vi "CHS_Teleop_System_CalcDriveMode.vi"(4 "Abs Traj 2":bool, 6 "Abs Traj 1":bool, 8 "Traj Rev Follow Orient":bool, 9 "Traj Rev Same Orient":bool, 10 "Traj Fwd Follow Orient":bool, 11 "Traj Fwd Same Orient":bool) -> (2 "Dirve Mode Changed":bool, 3 "Drive Mode":i32)   [LabVIEW 2019]
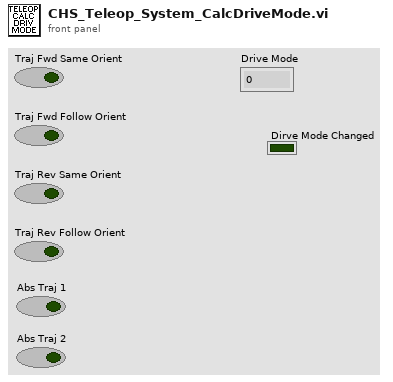
[diagram p1: front panel]
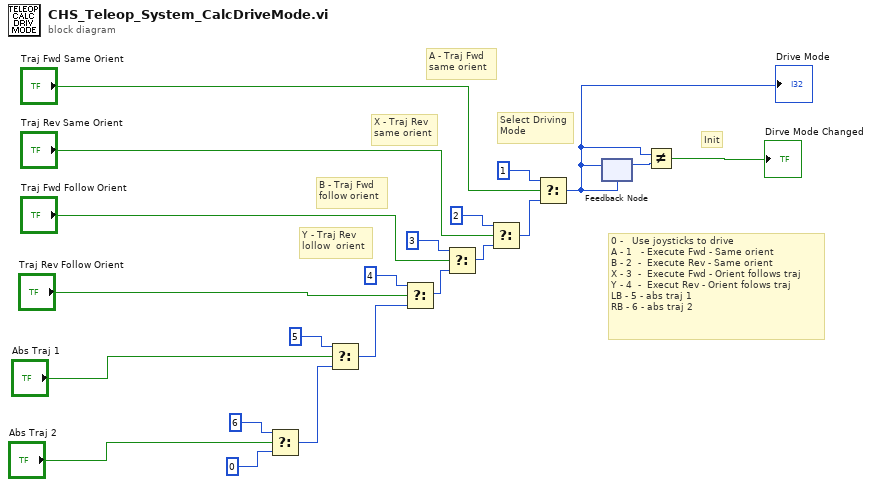
[diagram p0: block diagram]
diagram:
  # "0 -   Use joysticks to drive\nA - 1   - Execute Fwd - Same orient\nB - 2  -  Execute Rev - Same orient\nX - 3  -  Execute Fwd - Orient follows traj\nY - 4  -  Execut Rev - Orient folows traj\nLB - 5 - abs traj 1\nRB - 6 - abs traj 2"
  # "Init"
  # "Y - Traj Rev \nlollow  orient"
  # "B - Traj Fwd \nfollow orient"
  # "X - Traj Rev\nsame orient"
  # "A - Traj Fwd \nsame orient"
  # "Select Driving\nMode"
  n1 = Select(t=6, s="Abs Traj 2", f=0) -> (s? t:f=w3:i32)
  n2 = Select(t=5, s="Abs Traj 1", f=w3) -> (s? t:f=w4:i32)
  n3 = Select(t=4, s="Traj Rev Follow Orient", f=w4) -> (s? t:f=w18:i32)
  n4 = Select(t=3, s="Traj Fwd Follow Orient", f=w18) -> (s? t:f=w17:i32)
  n5 = Select(t=2, s="Traj Rev Same Orient", f=w17) -> (s? t:f=w14:i32)
  n6 = Select(t=1, s="Traj Fwd Same Orient", f=w14) -> (s? t:f=w11:i32)
  "Drive Mode" <- w11
  n7 = feedback #1(w11) -> (w10:i32)
  n8 = feedback-in #1(w11) -> ()
  n9 = Not Equal?(x=w11, y=w10) -> (x != y?=→"Dirve Mode Changed":bool)
